vi "Global Var.vi"() -> ()   [LabVIEW 2019]
panel:
  in  "Set X":dbl
  in  "Line Dis X":bool
  in  "Servo_Arm_Kick_main":bool
  in  "Servo_Camera_main":bool
  out "Time":dbl
  in  "Speed Low":bool
  out "Place_pos":dbl
  out "Place 3":dbl
  out "Place 2":dbl
  out "Place 1":dbl
  in  "BlueBox (yellow)":i16
  in  "BlueBox (blue)":i16
  in  "BlueBox (red)":i16
  in  "RedBox (yellow)":i16
  in  "RedBox (blue)":i16
  in  "RedBox (red)":i16
  in  "Stock":i16
  in  "BlueBox":i16
  in  "RedBox":i16=7
  in  "Color Box":u32(colorbox)
  in  "Qrcode":i16
  in  "GoalT/F":bool
  in  "Error theta 2":dbl=1.0
  in  "Error robot 2":dbl=0.1
  in  "QRCodeTick":bool
  in  "Servo Kick 2":u8(slide)=255 scale=255.0..200.0
  in  "Yellow No":string
  out "Cross Line Position":dbl
  in  "Set Y":dbl
  out "Limit Gripper":bool
  out "Vision Mode":i16
  in  "Zone":string
  in  "Color":string
  out "Image_line":T1(plugin-control)
  in  "Error Angle Line":dbl=0.10000000000000003
  out "Theta_line":bool
  out "Angle_Line":dbl
  out "X_Line":dbl
  in  "Status":string
  out "JPulse":bool
  in  "Line_X0":dbl(slide)=220.0 scale=210.0..250.0
  in  "Theta_set":dbl(slide) scale=-180.0..180.0
  in  "Y_set":dbl(slide) scale=-1.0..1.0
  in  "X_set":dbl(slide) scale=-1.0..1.0
  in  "Servo Kick":u8(slide)=200 scale=0.0..200.0
  in  "Servo Gripper":u8(slide)=100 scale=10.0..200.0
  in  "Servo Arm Kick":u8(slide)=30 scale=30.0..150.0
  in  "Servo socket":u8(slide)=100 scale=100.0..240.0
  in  "Servo Camera":u8(slide)=10 scale=0.0..200.0
  in  "Error Distance":dbl=12.0
  in  "Cross set":dbl=350.0
  in  "Error line":dbl=12.0
  in  "Error theta":dbl=1.0
  in  "Error robot":dbl=0.01
  in  "Line Dis":bool
  in  "Mode PID":bool
  in  "Motor_slide2":bool
  in  "Motor_slide1":bool
  in  "Motor_rotate":bool
  in  "LED camera":bool
  out "Theta_en":dbl
  out "Y_en":dbl
  out "X_en":dbl
  out "distance_sensor":dbl
  in  "Line_sensor":dbl(slide) scale=0.0..5.0
  out "Encoder 3":i32
  out "Encoder 2":i32
  out "Encoder 1":i32
  out "Speed(rpm) 3":i16
  out "Speed(rpm) 2":i16
  out "Speed(rpm) 1":i16
  out "Speed(rad/s) 3":dbl
  out "Speed(rad/s) 2":dbl
  out "Speed(rad/s) 1":dbl
  in  "INSpeed 3":dbl
  in  "INSpeed 2":dbl
  in  "INSpeed 1":dbl
  out "Status_line":bool
  out "Status_Distance":bool
  out "Status_theta":bool
  out "Status_x":bool
  out "Status_y":bool
  out "Start_SW":bool
  in  "Reset":bool=TRUE
  in  "ENA":bool=TRUE
  in  "Stop":bool
  # "Place 1"
  # "Place 2"
  # "Place 3"
  # "now position"
  # "ขึ้นสุด 0 ลงสุด 200 กลาง 110"
  # "285"
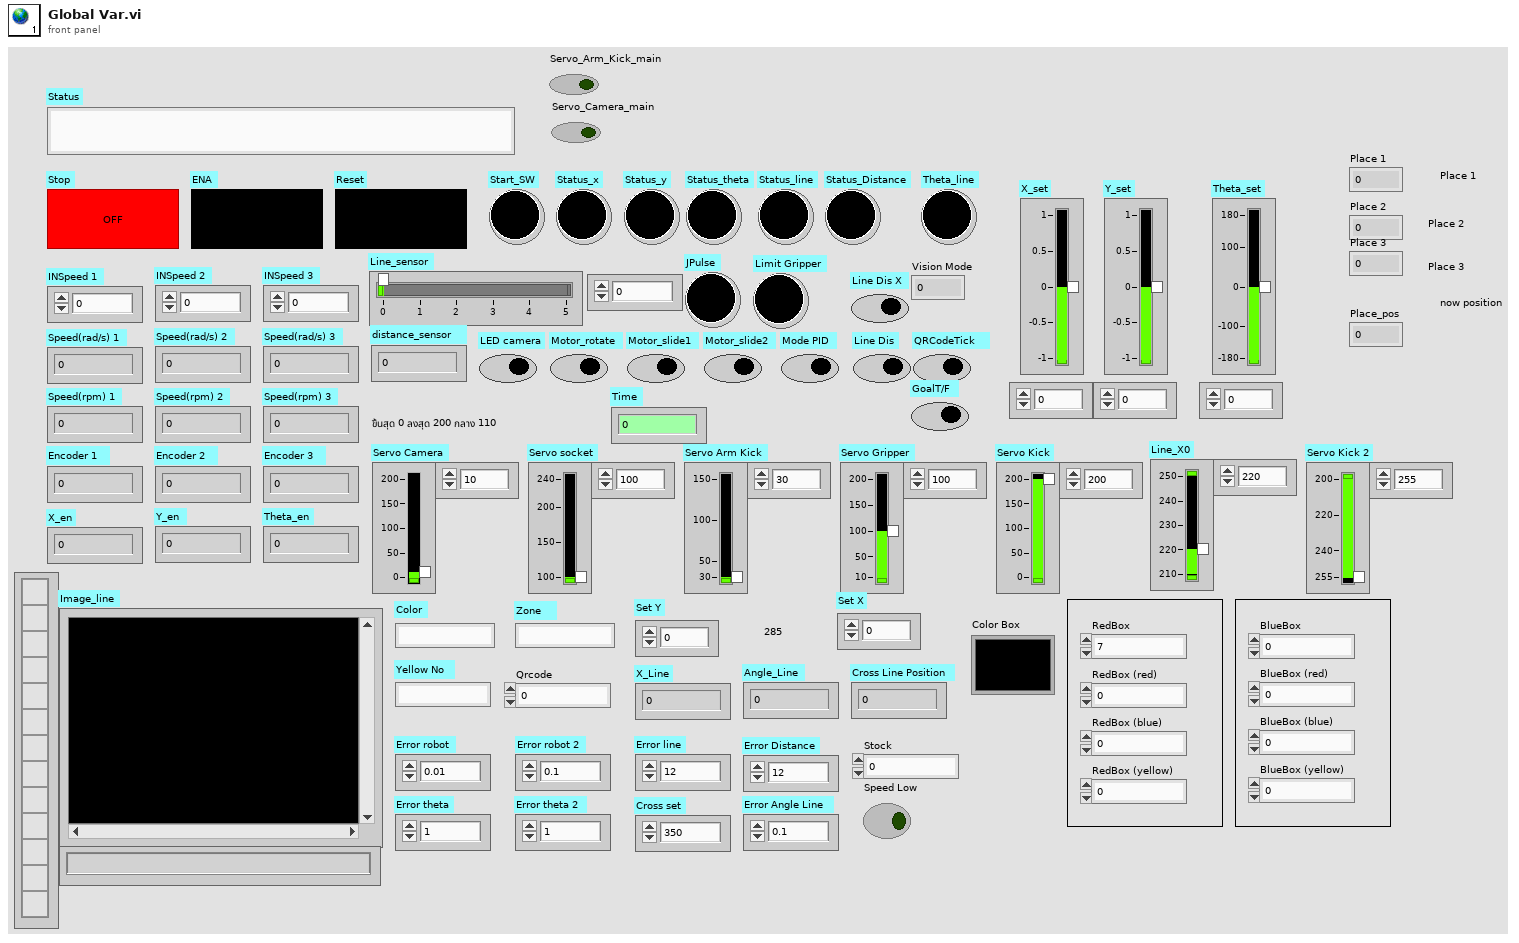
[diagram p1: front panel]
types:
  T1 = typedef "IMAQ Image.ctl" = refnum<image>
diagram:
